vi "FTW-Test-JSON-FloatingPoint.vi"() -> (0 "Test Result":errorcluster)   [LabVIEW 2014]
uses:
  src/core/json/FTW-JSON-Type.ctl
  src/core/error/FTW-ERR-Assert-DeveloperError.vi
  src/core/error/FTW-ERR-ThrowError.vi
  src/core/error/FTW-ERR-CallChain.vi
  src/core/string/FTW-STR-ReplaceWhitespace.vi
panel:
  out "JSON String (UTF-8)":string
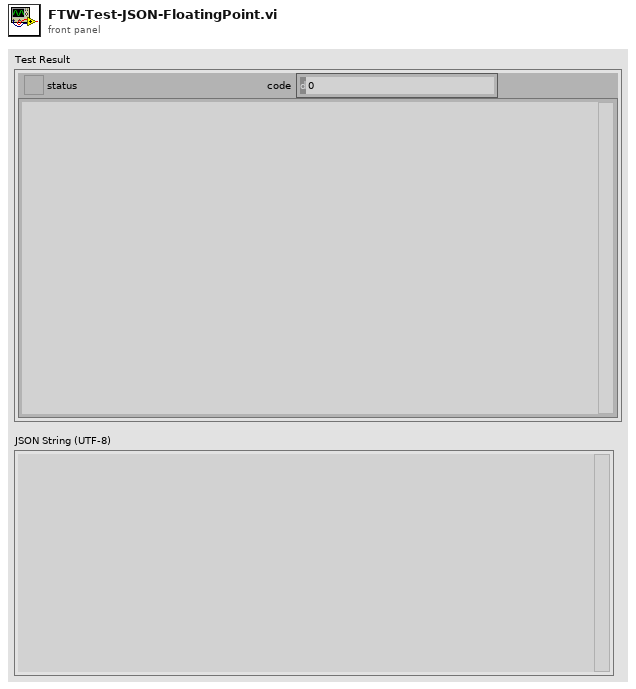
[diagram p1: front panel]
types:
  T1 = typedef "FTW-JSON-Type.ctl" = enum8{"Not Found", "Object", "Array", "String", "Number", "Boolean", "null"}
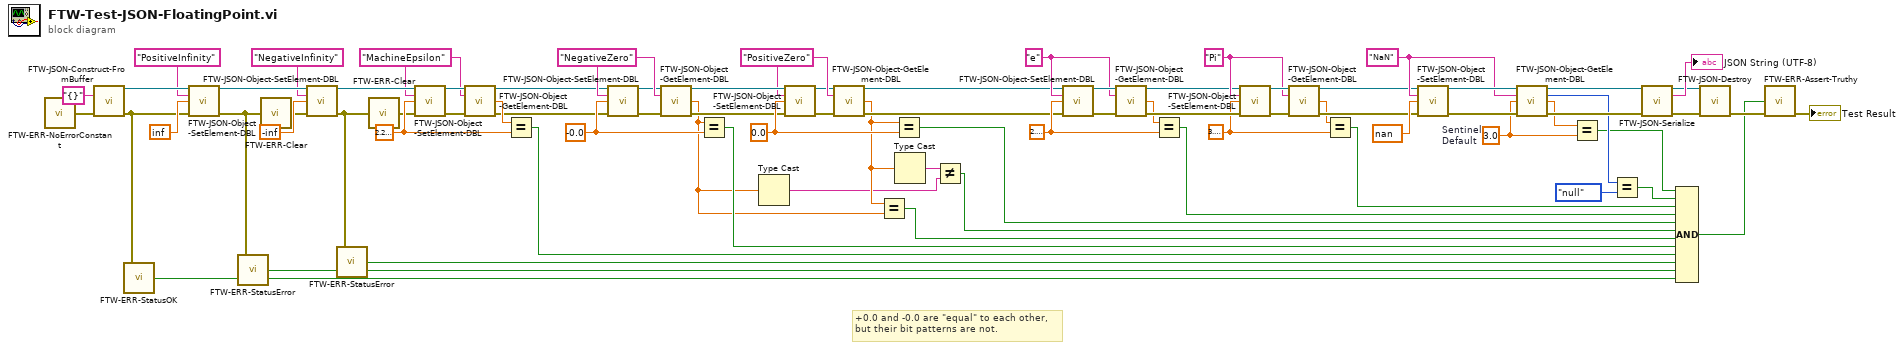
[diagram p0: block diagram]
diagram:
  w22 = 0.0
  w17 = "PositiveZero" ("Key")
  w15 = "NegativeZero" ("Key")
  w21 = -0.0
  w24 = 3.0  # Sentinel Default
  w41 = 3.141592653589793
  w52 = "Pi" ("Key")
  w54 = "e" ("Key")
  w57 = "NaN" ("Key")
  w43 = 2.718281828459045
  w62 = 2.220446049250313e-16
  w64 = "MachineEpsilon" ("Key")
  # "+0.0 and -0.0 are \"equal\" to each other,\nbut their bit patterns are not."
  n1 = call "FTW-ERR-NoErrorConstant.vi"() -> ("no error"=w78:errorcluster)
  n2 = call "FTW-JSON-Construct-FromBuffer.vi"("JSON String (UTF-8)"="{}", "error in"=w78) -> ("JSON Object"=w77:refnum<data-value>, "error out"=w36:errorcluster)  [unwired: 12 in]
  n3 = call "FTW-ERR-StatusOK.vi"("error to check"=w36) -> ("Status OK?"=w29:bool)
  n4 = call "FTW-JSON-Object-SetElement-DBL.vi"("JSON Object"=w77, "Key"="PositiveInfinity", "Value"=inf, "error in"=w36) -> ("JSON Object out"=w74:refnum<data-value>, "error out"=w35:errorcluster)  [unwired: 10 in]
  n5 = call "FTW-ERR-StatusError.vi"("error to check"=w35) -> ("Error?"=w30:bool)
  n6 = call "FTW-ERR-Clear.vi"("error to snuff"=w35) -> ("no error"=w34:errorcluster)
  n7 = call "FTW-JSON-Object-SetElement-DBL.vi"("JSON Object"=w74, "Key"="NegativeInfinity", "Value"=-inf, "error in"=w34) -> ("JSON Object out"=w71:refnum<data-value>, "error out"=w32:errorcluster)  [unwired: 10 in]
  n8 = call "FTW-ERR-StatusError.vi"("error to check"=w32) -> ("Error?"=w31:bool)
  n9 = call "FTW-ERR-Clear.vi"("error to snuff"=w32) -> ("no error"=w33:errorcluster)
  n10 = call "FTW-JSON-Object-SetElement-DBL.vi"("JSON Object"=w71, "Key"=w64, "Value"=w62, "error in"=w33) -> ("JSON Object out"=w65:refnum<data-value>, "error out"=w66:errorcluster)  [unwired: 10 in]
  n11 = call "FTW-JSON-Object-GetElement-DBL.vi"("JSON Object"=w65, "Key"=w64, "error in"=w66) -> ("JSON Object out"=w12:refnum<data-value>, "Value"=w63:dbl, "error out"=w10:errorcluster)  [unwired: 9 in, 1 out]
  n12 = Equal?(x=w63, y=w62) -> (x = y?=w37:bool)
  n13 = call "FTW-JSON-Object-SetElement-DBL.vi"("JSON Object"=w12, "Key"=w15, "Value"=w21, "error in"=w10) -> ("JSON Object out"=w13:refnum<data-value>, "error out"=w14:errorcluster)  [unwired: 10 in]
  n14 = call "FTW-JSON-Object-GetElement-DBL.vi"("JSON Object"=w13, "Key"=w15, "error in"=w14) -> ("JSON Object out"=w18:refnum<data-value>, "Value"=w5:dbl, "error out"=w20:errorcluster)  [unwired: 9 in, 1 out]
  n15 = Equal?(x=w5, y=w21) -> (x = y?=w8:bool)
  n16 = Type Cast(x=w5) -> (*(type *) &x=w2:string)  [unwired: 1 in]
  n17 = call "FTW-JSON-Object-SetElement-DBL.vi"("JSON Object"=w18, "Key"=w17, "Value"=w22, "error in"=w20) -> ("JSON Object out"=w16:refnum<data-value>, "error out"=w19:errorcluster)  [unwired: 10 in]
  n18 = call "FTW-JSON-Object-GetElement-DBL.vi"("JSON Object"=w16, "Key"=w17, "error in"=w19) -> ("JSON Object out"=w11:refnum<data-value>, "Value"=w4:dbl, "error out"=w9:errorcluster)  [unwired: 9 in, 1 out]
  n19 = Equal?(x=w4, y=w5) -> (x = y?=w6:bool)
  n20 = Equal?(x=w4, y=w22) -> (x = y?=w7:bool)
  n21 = Type Cast(x=w4) -> (*(type *) &x=w3:string)  [unwired: 1 in]
  n22 = Not Equal?(x=w3, y=w2) -> (x != y?=w1:bool)
  n23 = call "FTW-JSON-Object-SetElement-DBL.vi"("JSON Object"=w11, "Key"=w54, "Value"=w43, "error in"=w9) -> ("JSON Object out"=w56:refnum<data-value>, "error out"=w55:errorcluster)  [unwired: 10 in]
  n24 = call "FTW-JSON-Object-GetElement-DBL.vi"("JSON Object"=w56, "Key"=w54, "error in"=w55) -> ("JSON Object out"=w51:refnum<data-value>, "Value"=w44:dbl, "error out"=w45:errorcluster)  [unwired: 9 in, 1 out]
  n25 = Equal?(x=w44, y=w43) -> (x = y?=w38:bool)
  n26 = call "FTW-JSON-Object-SetElement-DBL.vi"("JSON Object"=w51, "Key"=w52, "Value"=w41, "error in"=w45) -> ("JSON Object out"=w53:refnum<data-value>, "error out"=w46:errorcluster)  [unwired: 10 in]
  n27 = call "FTW-JSON-Object-GetElement-DBL.vi"("JSON Object"=w53, "Key"=w52, "error in"=w46) -> ("JSON Object out"=w50:refnum<data-value>, "Value"=w42:dbl, "error out"=w49:errorcluster)  [unwired: 9 in, 1 out]
  n28 = Equal?(x=w42, y=w41) -> (x = y?=w40:bool)
  n29 = call "FTW-JSON-Object-SetElement-DBL.vi"("JSON Object"=w50, "Key"=w57, "Value"=nan, "error in"=w49) -> ("JSON Object out"=w59:refnum<data-value>, "error out"=w58:errorcluster)  [unwired: 10 in]
  n30 = call "FTW-JSON-Object-GetElement-DBL.vi"("JSON Object"=w59, "Key"=w57, "Default Value"=w24, "error in"=w58) -> ("JSON Object out"=w48:refnum<data-value>, "JSON Element Type"=w28:T1, "Value"=w25:dbl, "error out"=w47:errorcluster)  [unwired: 8 in]
  n31 = Equal?(x=w25, y=w24) -> (x = y?=w23:bool)
  n32 = Equal?(x=w28, y=FTW-JSON-Type."null") -> (x = y?=w26:bool)
  n33 = call "FTW-JSON-Serialize.vi"("JSON Object"=w48, "error in"=w47) -> ("JSON Object out"=w68:refnum<data-value>, "JSON String (UTF-8)"=→"JSON String (UTF-8)":string, "error out"=w67:errorcluster)  [unwired: 11 in]
  n34 = Compound Arithmetic op=AND(w23, w26, w40, w38, w7, w1, w6, w8, w37, w31, w30, w29) -> (w39:bool)
  n35 = call "FTW-JSON-Destroy.vi"("JSON Object"=w68, "error in"=w67) -> ("error out"=w61:errorcluster)  [unwired: 13 in]
  n36 = call "FTW-ERR-Assert-Truthy.vi"("Expected Truthy"=w39, "error in"=w61) -> ("error out"=→"Test Result":errorcluster)  [unwired: 13 in]
